vi "GE 5565PIORC.Registers.PCI Header Type.Configuration Layout Type.Get.vi"(8 "error in (no error)":errorcluster, 11 "GE 5565PIORC in":refnum<class "GE 5565PIORC.lvclass">) -> (0 "error out":errorcluster, 2 "Configuration Layout Type":u8, 3 "GE 5565PIORC out":refnum<class "GE 5565PIORC.lvclass">)   [LabVIEW 2016, in "GE 5565PIORC.lvclass"]
doc: "Specifies layout of bits $10 through $3F in Configuration Space. Only one encoding, $0, is defined. All other encodings are reserved."
uses:
  GE 5565PIORC.lvclass
  GE 5565PIORC.Registers.PCI Configuration.ctl
  GE 5565PIORC.lvclass/GE 5565PIORC.ctl
  GE 5565PIORC.Registers.PCI Configuration.Read (U8).vi
  GE 5565PIORC.Registers.Read.vi
  GE 5565PIORC.Registers.Read (U8).vi
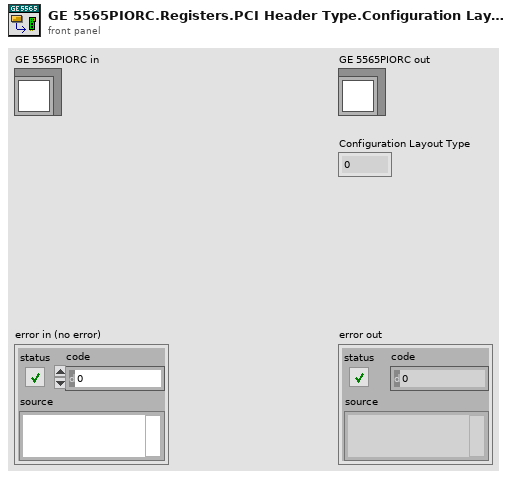
[diagram p1: front panel]
types:
  T1 = typedef "GE 5565PIORC.lvclass/GE 5565PIORC.Registers.PCI Configuration.ctl" = u32
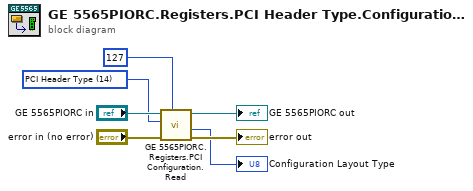
[diagram p0: block diagram]
diagram:
  w3 = T1 14 items=["PCI Configuration ID"=0, "PCI Command"=4, "PCI Status"=6, "PCI Revision ID"=8, "PCI Class Code"=9, "PCI Cache Line Size"=12, "PCI Latency Timer"=13, "PCI Header Type"=14, "PCI Built-in Self Test"=15, "PCIBAR0"=16, "PCIBAR1"=20, "PCIBAR2"=24, "PCIBAR3"=28, "PCIBAR4"=32, "PCIBAR5"=36, "PCI Cardbus CIS Pointer"=40, "PCI Subsystem Vendor ID"=44, "PCI Subsystem ID"=46, "PCI Expansion ROM Base"=48, "Capability Pointer"=52, "PCI Interrupt Line"=60, "PCI Interrupt Pin"=61, "PCI Min_Gnt"=62, "PCI Max_Lat"=63] ("PCI Configuration Registers")
  n1 = call-poly "GE 5565PIORC.Registers.PCI Configuration.Read.vi"("Mask (0xFF)"=u8 127 ("y"), "error in (no error)"="error in (no error)", "Register"=w3, "GE 5565PIORC in"="GE 5565PIORC in") -> ("error out"=→"error out":errorcluster, "Value"=→"Configuration Layout Type":u8, "GE 5565PIORC out"=→"GE 5565PIORC out":refnum<class "GE 5565PIORC.lvclass">)  [unwired: 5 in]
